vi "YAML_csv_entry.vi"(1 "value":string, 2 "name":string) -> (0 "result":string)   [LabVIEW 2011]
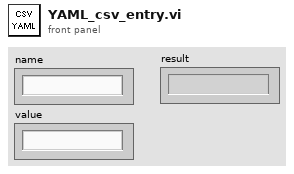
[diagram p1: front panel]
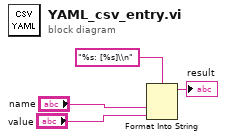
[diagram p0: block diagram]
diagram:
  n1 = Format Into String(format string="%s: [%s]\\n", "name", "value") -> (resulting string=→"result":string)  [unwired: 2 in, 1 out]
